vi "get_serviceType.vi"(0 "HGF_DIMServiceInfo":refnum<class "HGF_DIMSubscriber.lvclass">, 5 "error in (no error)":errorcluster) -> (13 "stamped":bool, 14 "dup HGF_DIMServiceInfo":refnum<class "HGF_DIMSubscriber.lvclass">, 17 "timeout [s]":i32, 18 "typeOfDimService":T1=4 items=["ONCE_ONLY"=1, "TIMED"=2, "MONITORED"=4], 19 "error out":errorcluster)   [LabVIEW 2012, in "HGF_DIM.lvlib" / "HGF_DIMSubscriber.lvclass"]
uses:
  HGF_DIMSubscriber.lvclass
  DimLVEvent/LVDimInterface/LVDimInterface.dim service type.ctl
  HGF_DIMSubscriber.lvclass/HGF_DIMSubscriber.ctl
  DimLVEvent/LVDimInterface/LVDimInterface.lvlib
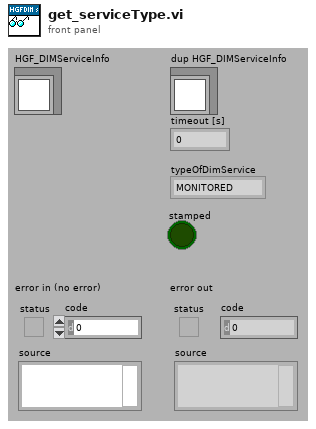
[diagram p1: front panel]
types:
  T1 = typedef "LVDimInterface.lvlib/LVDimInterface.dim service type.ctl" = u16
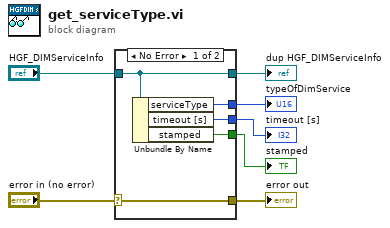
[diagram p0: block diagram]
diagram:
  n1 = case shown="No Error" "error in (no error)" {
    selector: "error in (no error)" -> [w12 w13]
    tunnel: [w12 w13] -> w6
    tunnel: [w11 w14] -> w4
    tunnel: "HGF_DIMServiceInfo" -> [w11 w14]
    tunnel: [w10 _] -> w3
    tunnel: [w9 _] -> w2
    tunnel: [w8 _] -> w1
    frame No Error {
      n2 = Unbundle By Name(w11) -> ("serviceType"=w10:T1, "timeout [s]"=w9:i32, "stamped"=w8:bool)
    }
    frame Error {
    }
  }
  "error out" <- w6
  "dup HGF_DIMServiceInfo" <- w4
  "typeOfDimService" <- w3
  "timeout [s]" <- w2
  "stamped" <- w1
